vi "Fail If Equal.vi"(6 "Delta":variant, 7 "Description":string, 8 "error in (no error)":errorcluster, 9 "Actual":variant, 10 "Expected":variant, 11 "LUnit Test Case In":refnum<class "LUnit Test Case V2.lvclass">) -> (0 "error out":errorcluster, 3 "LUnit Test Case Out":refnum<class "LUnit Test Case V2.lvclass">)   [LabVIEW 2020, in "LUnit Test Case V2.lvclass"]
doc: "***DEPRECATED*** Use the maleable (.vim) version of this VI instead. \n\nGenerates a fail result for the calling test method if the inputs are equal. For numeric inputs, a tolerance range may be specified using the Delta input. A description may be provided to the result."
uses:
  LUnit Test Case V2.lvclass
  LUnit Test Case V2.lvclass/LUnit Test Case V2.ctl
  7d9af9d3-0d3f-4211-9f2d-a5e09b8a4e0e.vi
  Fail.vi
  Pass.vi
  Private/Compare Variants.vi
  Private/Describe Comparison.vi
  Private/Append Result.vi
  Private/Variant to string.vi
  <vilib>/Utility/Data Type/Get Type Information.vi
  <vilib>/Utility/LVClass/Get LV Class Name.vi
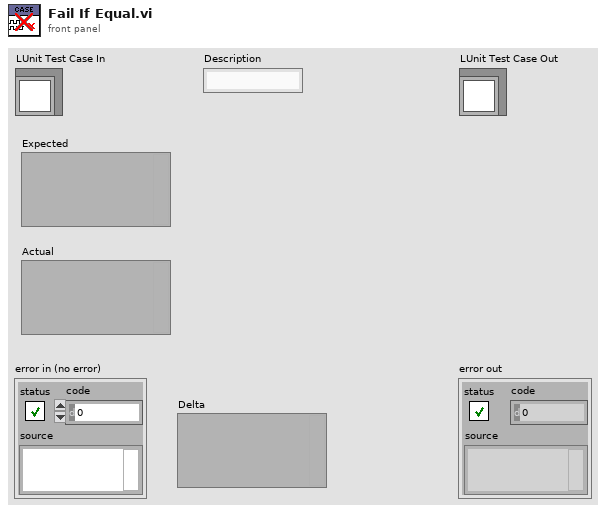
[diagram p1: front panel]
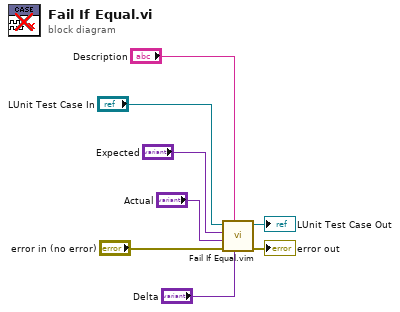
[diagram p0: block diagram]
diagram:
  n1 = call "Fail If Equal.vim"("Delta"="Delta", "Description"="Description", "error in (no error)"="error in (no error)", "Actual"="Actual", "Expected"="Expected", "LUnit Test Case In"="LUnit Test Case In") -> ("error out"=→"error out":errorcluster, "LUnit Test Case Out"=→"LUnit Test Case Out":refnum<class "LUnit Test Case V2.lvclass">)  [unwired: 4 in]
